vi "TcM08-002_DevelopmentDistribution.vi"(1 "Input buffer":T3="1", 3 "Invocation info":T2, 5 "error in (no error)":errorcluster, 6 "Add log to result?":bool) -> (16 "Test Data":T1 {"Numeric Measurement" format="%.2f"}, 19 "error out":errorcluster)   [LabVIEW 2009]
doc: "Test case template."
uses:
  Shared/Support_InputBuffer.ctl
  Shared/Support_InvocationInfo.ctl
  Shared/Support_TestData.ctl
panel:
  in  "Test name":string="TcM08-002 Development distribution"
  out "Test result":bool
  out "Result":string
  # "Verify that a LabVIEW application can be saved as a \ndevelopement distribution if all dynamically called\nmethod is added to the llb."
  # "Sub test case"
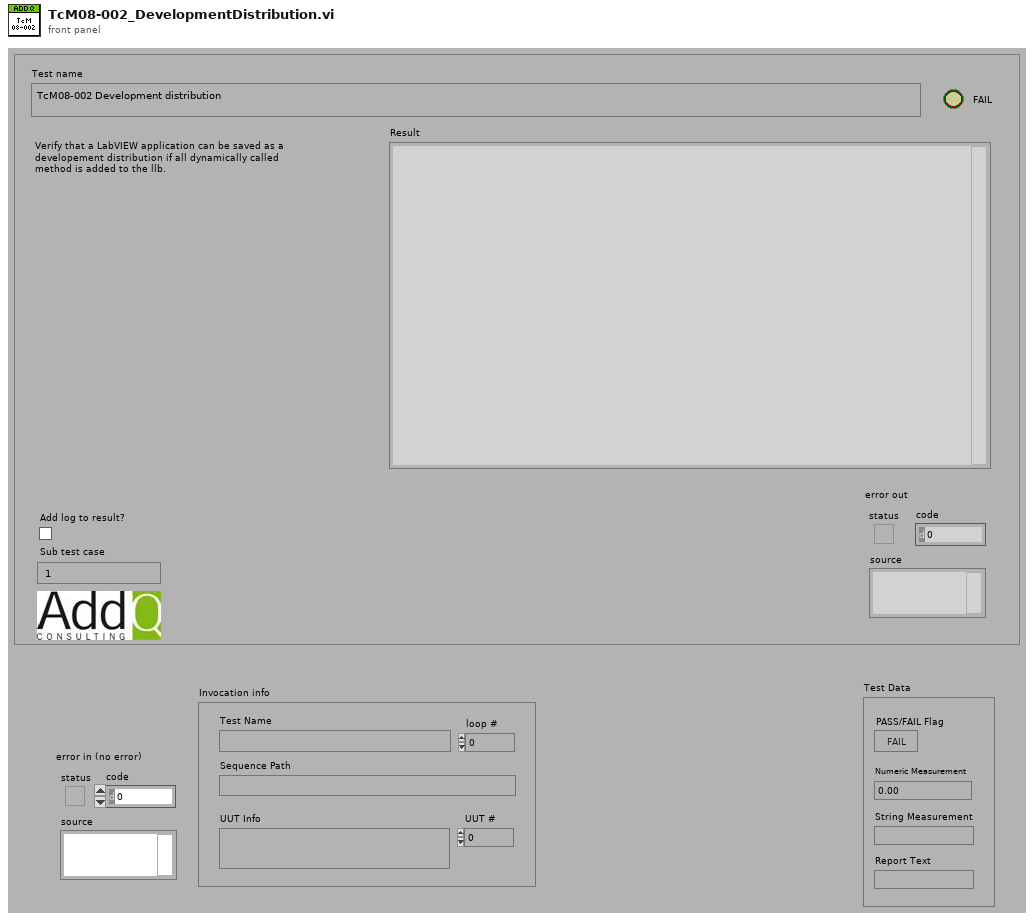
[diagram p1: front panel]
types:
  T1 = typedef "Support_TestData.ctl" = cluster{"PASS/FAIL Flag":bool, "Numeric Measurement":dbl, "String Measurement":string, "Report Text":string}
  T2 = typedef "Support_InvocationInfo.ctl" = cluster{"UUT #":i32, "loop #":i32, "UUT Info":string, "Test Name":string, "Sequence Path":path}
  T3 = typedef "Support_InputBuffer.ctl" = string
  T4 = typedef "Support_ResultType.ctl" = cluster{"Pass":bool, "Comment":string, "MeasurementValue":dbl}
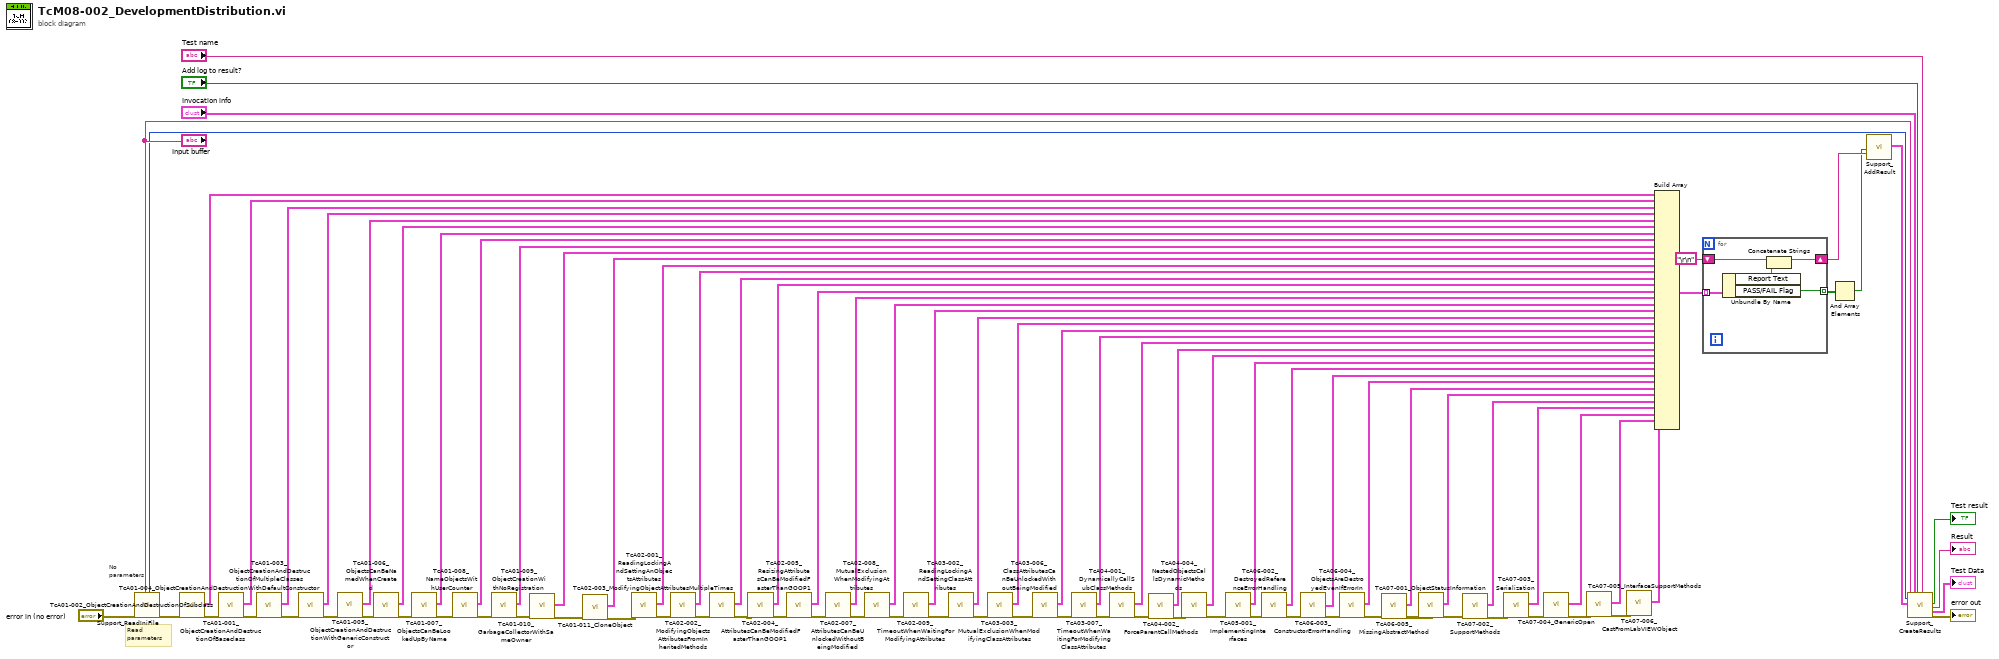
[diagram p0: block diagram]
diagram:
  # "No\nparameters"
  # "Read\nparameters"
  n1 = call "Support_ReadIniFile.vi"("error in (no error)"="error in (no error)", "Sub test case"="Input buffer") -> ("Timer start"=w80:u32, "error out"=w46:errorcluster)  [unwired: 10 in, 6 out]
  n2 = call "TcA01-001_ObjectCreationAndDestructionOfBaseclass.vi"("error in (no error)"=w46) -> ("Test Data"=w44:T1, "error out"=w45:errorcluster)  [unwired: 17 in]
  n3 = call "TcA01-002_ObjectCreationAndDestructionOfSubclass.vi"("error in (no error)"=w45) -> ("Test Data"=w69:T1, "error out"=w79:errorcluster)  [unwired: 17 in]
  n4 = call "TcA01-003_ObjectCreationAndDestructionOfMultipleClasses.vi"("error in (no error)"=w79) -> ("Test Data"=w68:T1, "error out"=w33:errorcluster)  [unwired: 17 in]
  n5 = call "TcA01-004_ObjectCreationAndDestructionWithDefaultConstructor.vi"("error in (no error)"=w33) -> ("Test Data"=w31:T1, "error out"=w32:errorcluster)  [unwired: 17 in]
  n6 = call "TcA01-005_ObjectCreationAndDestructionWithGenericConstructor.vi"("error in (no error)"=w32) -> ("Test Data"=w30:T1, "error out"=w28:errorcluster)  [unwired: 17 in]
  n7 = call "TcA01-006_ObjectsCanBeNamedWhenCreated.vi"("error in (no error)"=w28) -> ("Test Data"=w29:T1, "error out"=w78:errorcluster)  [unwired: 17 in]
  n8 = call "TcA01-007_ObjectsCanBeLookedUpByName.vi"("error in (no error)"=w78) -> ("Test Data"=w67:T1, "error out"=w39:errorcluster)  [unwired: 17 in]
  n9 = call "TcA01-008_NameObjectsWithUserCounter.vi"("error in (no error)"=w39) -> ("Test Data"=w38:T1, "error out"=w21:errorcluster)  [unwired: 17 in]
  n10 = call "TcA01-009_ObjectCreationWithNoRegistration.vi"("error in (no error)"=w21) -> ("Test Data"=w20:T1, "error out"=w10:errorcluster)  [unwired: 17 in]
  n11 = call "TcA01-010_GarbageCollectorWithSameOwner.vi"("error in (no error)"=w10) -> ("Test Data"=w9:T1, "error out"=w7:errorcluster)  [unwired: 17 in]
  n12 = call "TcA01-011_CloneObject.vi"("error in (no error)"=w7) -> ("Test Data"=w5:T1, "error out"=w6:errorcluster)  [unwired: 17 in]
  n13 = call "TcA02-001_ReadingLockingAndSettingAnObjectsAttributes.vi"("error in (no error)"=w6) -> ("Test Data"=w66:T1, "error out"=w43:errorcluster)  [unwired: 17 in]
  n14 = call "TcA02-002_ModifyingObjectsAttributesFromInheritedMethods.vi"("error in (no error)"=w43) -> ("Test Data"=w41:T1, "error out"=w42:errorcluster)  [unwired: 17 in]
  n15 = call "TcA02-003_ModifyingObjectAttributesMultipleTimes.vi"("error in (no error)"=w42) -> ("Test Data"=w65:T1, "error out"=w77:errorcluster)  [unwired: 17 in]
  n16 = call "TcA02-004_AttributesCanBeModifiedFasterThanGOOP1.vi"("error in (no error)"=w77) -> ("Test Data"=w64:T1, "error out"=w76:errorcluster)  [unwired: 17 in]
  n17 = call "TcA02-005_ResizingAttributesCanBeModifiedFasterThanGOOP1.vi"("error in (no error)"=w76) -> ("Test Data"=w63:T1, "error out"=w34:errorcluster)  [unwired: 17 in]
  n18 = call "TcA02-007_AttributesCanBeUnlockedWithoutBeingModified.vi"("error in (no error)"=w34) -> ("Test Data"=w62:T1, "error out"=w75:errorcluster)  [unwired: 17 in]
  n19 = call "TcA02-008_MutualExclusionWhenModifyingAttributes.vi"("error in (no error)"=w75) -> ("Test Data"=w61:T1, "error out"=w74:errorcluster)  [unwired: 17 in]
  n20 = call "TcA02-009_TimeoutWhenWaitingForModifyingAttributes.vi"("error in (no error)"=w74) -> ("Test Data"=w60:T1, "error out"=w35:errorcluster)  [unwired: 17 in]
  n21 = call "TcA03-002_ReadingLockingAndSettingClassAttributes.vi"("error in (no error)"=w35) -> ("Test Data"=w59:T1, "error out"=w73:errorcluster)  [unwired: 17 in]
  n22 = call "TcA03-003_MutualExclusionWhenModifyingClassAttributes.vi"("error in (no error)"=w73) -> ("Test Data"=w58:T1, "error out"=w37:errorcluster)  [unwired: 17 in]
  n23 = call "TcA03-006_ClassAttributesCanBeUnlockedWithoutBeingModified.vi"("error in (no error)"=w37) -> ("Test Data"=w57:T1, "error out"=w72:errorcluster)  [unwired: 17 in]
  n24 = call "TcA03-007_TimeoutWhenWaitingForModifyingClassAttributes.vi"("error in (no error)"=w72) -> ("Test Data"=w56:T1, "error out"=w36:errorcluster)  [unwired: 17 in]
  n25 = call "TcA04-001_DynamicallyCallSubClassMethods.vi"("error in (no error)"=w36) -> ("Test Data"=w55:T1, "error out"=w4:errorcluster)  [unwired: 17 in]
  n26 = call "TcA04-002_ForceParentCallMethods.vi"("error in (no error)"=w4) -> ("Test Data"=w1:T1, "error out"=w3:errorcluster)  [unwired: 17 in]
  n27 = call "TcA04-004_NestedObjectsCallsDynamicMethods.vi"("error in (no error)"=w3) -> ("Test Data"=w2:T1, "error out"=w19:errorcluster)  [unwired: 17 in]
  n28 = call "TcA05-001_ImplementingInterfaces.vi"("error in (no error)"=w19) -> ("Test Data"=w17:T1, "error out"=w18:errorcluster)  [unwired: 17 in]
  n29 = call "TcA06-002_DestroyedReferenceErrorHandling.vi"("error in (no error)"=w18) -> ("Test Data"=w54:T1, "error out"=w71:errorcluster)  [unwired: 17 in]
  n30 = call "TcA06-003_ConstructorErrorHandling.vi"("error in (no error)"=w71) -> ("Test Data"=w53:T1, "error out"=w70:errorcluster)  [unwired: 17 in]
  n31 = call "TcA06-004_ObjectsAreDestroyedEvenIfErrorIn.vi"("error in (no error)"=w70) -> ("Test Data"=w52:T1, "error out"=w16:errorcluster)  [unwired: 17 in]
  n32 = call "TcA06-005_MissingAbstractMethod.vi"("error in (no error)"=w16) -> ("Test Data"=w14:T1, "error out"=w15:errorcluster)  [unwired: 17 in]
  n33 = call "TcA07-001_ObjectStatusInformation.vi"("error in (no error)"=w15) -> ("Test Data"=w51:T1, "error out"=w27:errorcluster)  [unwired: 17 in]
  n34 = call "TcA07-002_SupportMethods.vi"("error in (no error)"=w27) -> ("Test Data"=w25:T1, "error out"=w26:errorcluster)  [unwired: 17 in]
  n35 = call "TcA07-003_Serialization.vi"("error in (no error)"=w26) -> ("Test Data"=w24:T1, "error out"=w23:errorcluster)  [unwired: 17 in]
  n36 = call "TcA07-004_GenericOpen.vi"("error in (no error)"=w23) -> ("Test Data"=w22:T1, "error out"=w13:errorcluster)  [unwired: 17 in]
  n37 = call "TcA07-005_InterfaceSupportMethods.vi"("error in (no error)"=w13) -> ("Test Data"=w12:T1, "error out"=w11:errorcluster)  [unwired: 17 in]
  n38 = call "TcA07-006_CastFromLabVIEWObject.vi"("error in (no error)"=w11) -> ("Test Data"=w8:T1)  [unwired: 17 in, 1 out]
  n39 = Build Array(w44, w69, w68, w31, w30, w29, w67, w38, w20, w9, w5, w66, w41, w65, w64, w63, w62, w61, w60, w59, w58, w57, w56, w55, w1, w2, w17, w54, w53, w52, w14, w51, w25, w24, w22, w12, w8) -> (w50:T1[])
  n40 = for {
    tunnel: w50 -> [w95] mode=indexing
    tunnel: [w94] -> w48 mode=indexing
    shift-right: [w91] -> w49
    shift-left: "\r\n" -> [w92]
    n41 = Unbundle By Name(w95) -> ("Report Text"=w93:string, "PASS/FAIL Flag"=w94:bool)
    n42 = Concatenate Strings(w92, w93) -> (w91:string)
  }
  n43 = And Array Elements(Boolean array=w48) -> (logical AND=w47:bool)
  n44 = call "Support_AddResult.vi"("Pass"=w47, "Comment"=w49) -> ("Results out"=w83:T4[])  [unwired: 17 in]
  n45 = call "Support_CreateResults.vi"("Sub test case"="Input buffer", "Timer start"=w80, "Results"=w83, "Invocation info"="Invocation info", "Add log to result?"="Add log to result?", "Test name"="Test name") -> ("Pass/fail flag"=→"Test result":bool, "Result"=→"Result":string, "Test Data"=→"Test Data":T1, "error out"=→"error out":errorcluster)  [unwired: 10 in]
